vi "Auto Loop 1.vi"(10 "auto #":u32, 11 "Call Context":T1) -> (0 "Loop 1 Value2":dbl, 1 "Loop 1 Value1":dbl, 2 "Loop 1 exit value":i32, 3 "Loop 1 SubState":T2=enum."auto")   [LabVIEW 2011]
uses:
  subStates.ctl
  <vilib>/Rock Robotics/WPI/DriverStation/WPI_DriverStationDerivedRobotMode.ctl
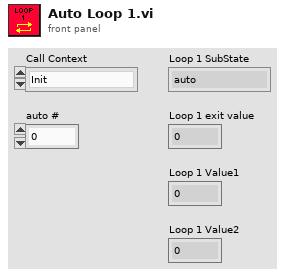
[diagram p1: front panel]
types:
  T1 = typedef "WPI_DriverStationDerivedRobotMode.ctl" = enum16{"Init", "Execute", "Stop"}
  T2 = typedef "subStates.ctl" = enum16{"null", "wait", "driver control", "auto", "manual override", "autoDrive", "hold position", "rotate", "end"}
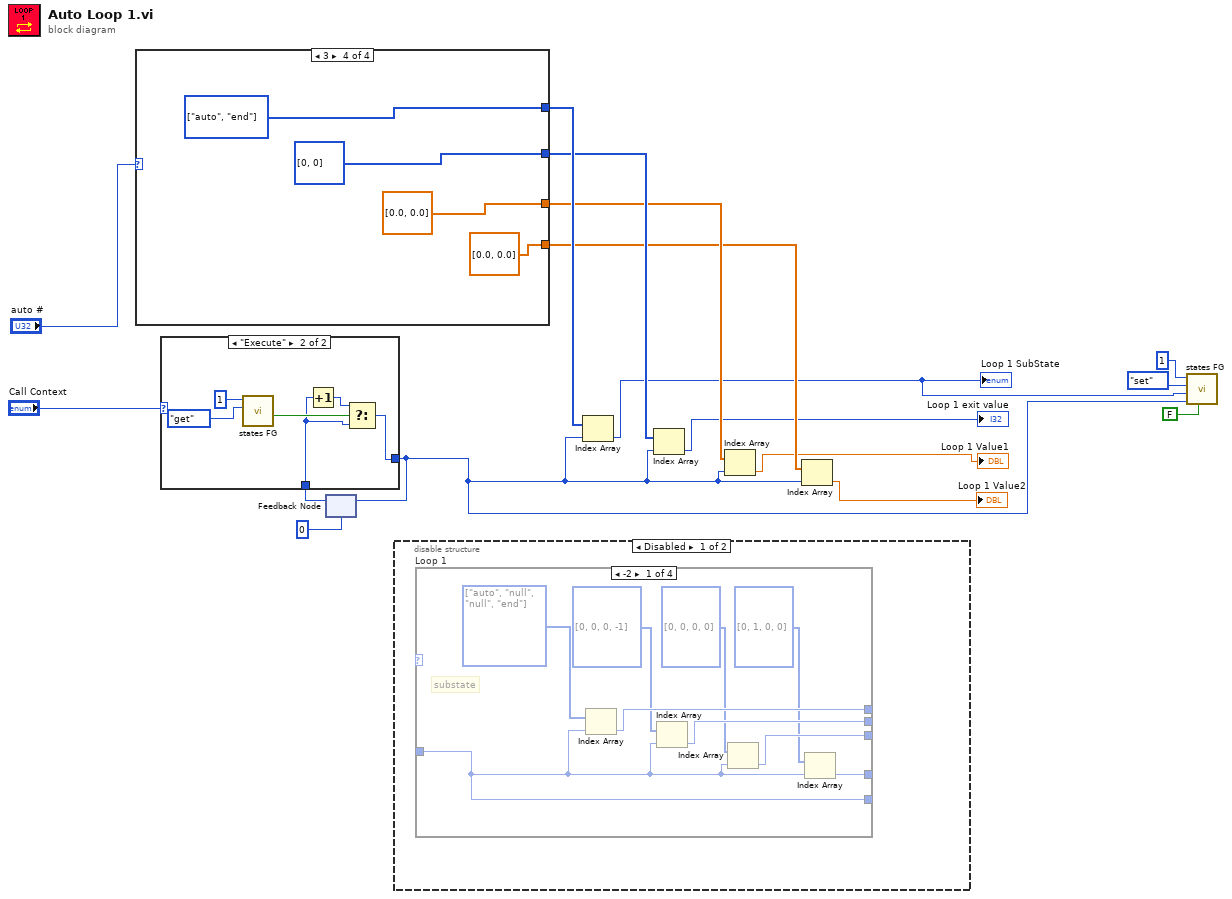
[diagram p0: block diagram]
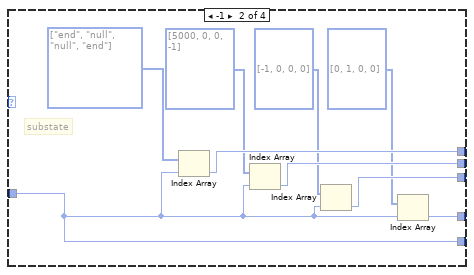
[diagram p2: hidden frame]
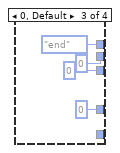
[diagram p3: hidden frame]
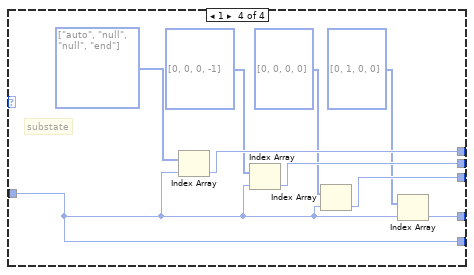
[diagram p4: hidden frame]
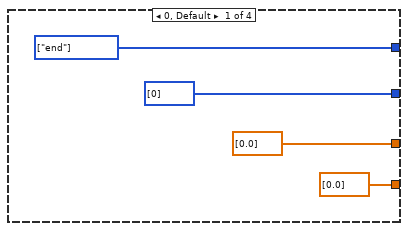
[diagram p6: hidden frame]
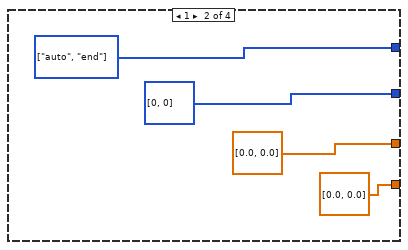
[diagram p7: hidden frame]
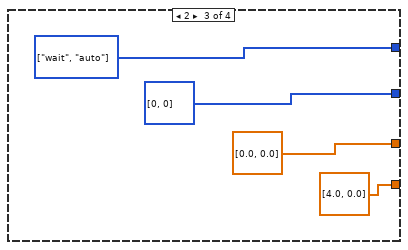
[diagram p8: hidden frame]
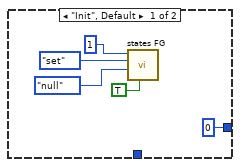
[diagram p9: hidden frame]
diagram:
  n1 = case shown="3" "auto #" {
    tunnel: [dbl[] [0.0] ("value2 array") dbl[] [0.0, 0.0] ("value2 array") dbl[] [4.0, 0.0] ("value2 array") dbl[] [0.0, 0.0] ("value2 array")] -> w8
    tunnel: [dbl[] [0.0] ("value1 array") dbl[] [0.0, 0.0] ("value1 array") dbl[] [0.0, 0.0] ("value1 array") dbl[] [0.0, 0.0] ("value1 array")] -> w9
    tunnel: [w18 w22 w26 w30] -> w11
    tunnel: [i32[] [0] ("exit value array") i32[] [0, 0] ("exit value array") i32[] [0, 0] ("exit value array") i32[] [0, 0] ("exit value array")] -> w10
    frame 0, Default {
      w18 = T2[] [enum."end"] items=["null", "wait", "driver control", "auto", "manual override", "autoDrive", "hold position", "rotate", "end"] ("substate array")
    }
    frame 1 {
      w22 = T2[] [enum."auto", enum."end"] items=["null", "wait", "driver control", "auto", "manual override", "autoDrive", "hold position", "rotate", "end"] ("substate array")
    }
    frame 2 {
      w26 = T2[] [enum."wait", enum."auto"] items=["null", "wait", "driver control", "auto", "manual override", "autoDrive", "hold position", "rotate", "end"] ("substate array")
    }
    frame 3 {
      w30 = T2[] [enum."auto", enum."end"] items=["null", "wait", "driver control", "auto", "manual override", "autoDrive", "hold position", "rotate", "end"] ("substate array")
    }
  }
  n2 = feedback #1(0 ("Value1 2")) -> (w13:i32)
  n3 = case shown="\"Execute\"" "Call Context" {
    tunnel: [0 ("Value1 2") w42] -> w2
    tunnel: w13 -> [_ w39]
    frame "Init", Default {
      n4 = call "states FG.vi"("exit in"=TRUE, "subState in"=subStates."null", "menu (get)"=enum16{"set", "get"}."set", "Loop ID"=1) -> ()  [unwired: 4 in, 4 out]
    }
    frame "Execute" {
      n5 = call "states FG.vi"("menu (get)"=enum16{"set", "get"}."get", "Loop ID"=1) -> ("exit out"=w41:bool)  [unwired: 6 in, 3 out]
      n6 = Increment(x=w39) -> (x+1=w43:i32)
      n7 = Select(t=w43, s=w41, f=w39) -> (s? t:f=w42:i32)
    }
  }
  n8 = feedback-in #1(w2) -> ()
  n9 = disable-structure shown="Disabled" {
    frame Disabled {
      n10 = case "Loop 1" shown="-2" {
        selector: _ -> [_ _ _ _]
        tunnel: _ -> [w44 w53 _ w66]
        tunnel: [w52 w61 subStates."end" ("Enum") w74] -> _
        tunnel: [w51 w60 0 ("Value1 2") w73] -> _
        tunnel: [w50 w59 0 ("Value1 2") w72] -> _
        tunnel: [w49 w58 0 ("Value1 2") w71] -> _
        tunnel: [w44 w53 _ w66] -> _
        frame -2 {
          w48 = T2[] [enum."auto", enum."null", enum."null", enum."end"] items=["null", "wait", "driver control", "auto", "manual override", "autoDrive", "hold position", "rotate", "end"] ("SubState Array")
          # "substate"
          n11 = Index Array(array=w48, index=w44) -> (element=w52:T2)
          n12 = Index Array(array=i32[] [0, 0, 0, -1], index=w44) -> (element=w51:i32)
          n13 = Index Array(array=i32[] [0, 0, 0, 0], index=w44) -> (element=w50:i32)
          n14 = Index Array(array=i32[] [0, 1, 0, 0], index=w44) -> (element=w49:i32)
        }
        frame -1 {
          w57 = T2[] [enum."end", enum."null", enum."null", enum."end"] items=["null", "wait", "driver control", "auto", "manual override", "autoDrive", "hold position", "rotate", "end"] ("SubState Array")
          # "substate"
          n15 = Index Array(array=w57, index=w53) -> (element=w61:T2)
          n16 = Index Array(array=i32[] [5000, 0, 0, -1], index=w53) -> (element=w60:i32)
          n17 = Index Array(array=i32[] [-1, 0, 0, 0], index=w53) -> (element=w59:i32)
          n18 = Index Array(array=i32[] [0, 1, 0, 0], index=w53) -> (element=w58:i32)
        }
        frame 0, Default {
        }
        frame 1 {
          w70 = T2[] [enum."auto", enum."null", enum."null", enum."end"] items=["null", "wait", "driver control", "auto", "manual override", "autoDrive", "hold position", "rotate", "end"] ("SubState Array")
          # "substate"
          n19 = Index Array(array=w70, index=w66) -> (element=w74:T2)
          n20 = Index Array(array=i32[] [0, 0, 0, -1], index=w66) -> (element=w73:i32)
          n21 = Index Array(array=i32[] [0, 0, 0, 0], index=w66) -> (element=w72:i32)
          n22 = Index Array(array=i32[] [0, 1, 0, 0], index=w66) -> (element=w71:i32)
        }
      }
    }
    frame Enabled {
    }
  }
  n23 = Index Array(array=w11, index=w2) -> (element=w1:T2)
  "Loop 1 SubState" <- w1
  n24 = Index Array(array=w10, index=w2) -> (element=→"Loop 1 exit value":i32)
  n25 = Index Array(array=w9, index=w2) -> (element=→"Loop 1 Value1":dbl)
  n26 = Index Array(array=w8, index=w2) -> (element=→"Loop 1 Value2":dbl)
  n27 = call "states FG.vi"("exit in"=FALSE, "state # in"=w2, "subState in"=w1, "menu (get)"=enum16{"set", "get"}."set", "Loop ID"=1) -> ()  [unwired: 3 in, 4 out]
